vi "turning code.vi"   [LabVIEW 2016]
uses:
  <vilib>/NXT/Block Support/NXT_OutputPort.ctl
  <vilib>/NXT/NXTIO Xnodes/NXTIONodeSubVIs/NXTStopMotors.vi
  <vilib>/NXT/NXTIO Xnodes/NXTIONodeSubVIs/NXTMoveMotors.vi
  <vilib>/NXT/NXTIO Xnodes/NXTIONodeSubVIs/NXTMotorRunDistance.vi
  <vilib>/NXT/Subs/LVHSConnector.ctl
  <vilib>/NXT/NXTIO Xnodes/AddressXNode/NXTIOAddress.xnode
  <vilib>/NXT/NXTIO Xnodes/NXTIOXNode/NXTIO.xnode
  <vilib>/NXT/LegoClasses/BrickReference/BrickReference.lvclass
types:
  T1 = typedef "NXT_OutputPort.ctl" = u8
  T2 = typedef "LVHSConnector.ctl" = refnum<class "BrickReference.lvclass">
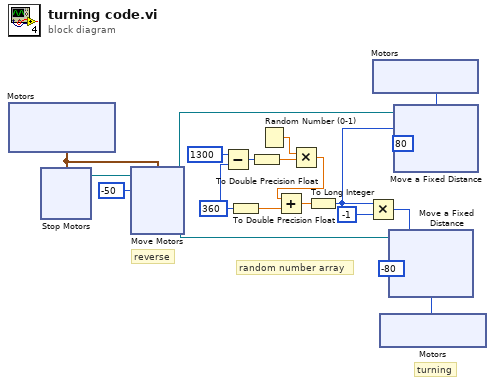
[diagram p0: block diagram]
diagram:
  w9 = 360
  # "turning"
  # "random number array"
  # "reverse"
  n1 = xnode "Motors"() -> ("Motor"=w17:cluster{"Port":T1, "Port":T1})
  n2 = xnode "Stop Motors"("Motors"=w17) -> ("NXT/EV3"=w19:T2)  [unwired: 1 in]
  n3 = xnode "Move Motors"("Power/Speed 1"=i8 -50, "Motors"=w17, "NXT/EV3"=w19) -> ("NXT/EV3"=w12:T2)  [unwired: 1 in]
  n4 = Subtract(x=1300, y=w9) -> (x-y=w10:i32)
  n5 = To Double Precision Float(number=w9) -> (double precision float=w8:dbl)
  n6 = To Double Precision Float(number=w10) -> (double precision float=w7:dbl)
  n7 = Random Number (0-1)() -> (number: 0 to 1=w6:dbl)
  n8 = Multiply(x=w6, y=w7) -> (x*y=w4:dbl)
  n9 = Add(x=w4, y=w8) -> (x+y=w5:dbl)
  n10 = To Long Integer(number=w5) -> (32bit integer=w3:i32)
  n11 = Multiply(x=w3, y=-1) -> (x*y=w1:i32)
  n12 = xnode "Motors"() -> ("Motor"=w16:T1)
  n13 = xnode "Motors"() -> ("Motor"=w15:T1)
  n14 = xnode "Move a Fixed Distance"("Speed 1"=i8 -80 ("Power/Speed 1"), "Distance 1"=w1, "Motors"=w15, "NXT/EV3"=w12) -> ()  [unwired: 1 out]
  n15 = xnode "Move a Fixed Distance"("Speed 1"=i8 80 ("Power/Speed 1"), "Distance 1"=w3, "Motors"=w16, "NXT/EV3"=w12) -> ()  [unwired: 1 out]
